vi "Send Finalize View Init.vi"(7 "Priority":T1=enum."Normal" caption="Message Priority (Normal)", 8 "error in (no error)":errorcluster, 10 "View Name":string, 11 "Message Enqueuer in":refnum<class "Message Enqueuer.lvclass">) -> (0 "error out":errorcluster, 3 "Message Enqueuer out":refnum<class "Message Enqueuer.lvclass">)   [LabVIEW 2023, in "Event Actors.lvlib" / "Finalize View Init Msg.lvclass"]
doc: "Sends the <b>Event Actors.lvlib:Finalize View Init Msg.lvclass</b> message.\n\nThis message will call <b>Finalize View Init.vi</b> on the <b>Event Actors.lvlib:Controller Actor.lvclass</b> actor.\n\n<b>Finalize View Init.vi Description</b>\nOverride this method to finalize Views' initialization by generating Controller events to the View specified in the \"View Name\" input terminal. To this end you can call the method \"Generate Event to View\". A typical use case is that of generating Controller events to update the Views upon init about the current state of the Controller."
uses:
  Finalize View Init Msg.lvclass
  Finalize View Init Msg.lvclass/Finalize View Init Msg.ctl
  <vilib>/ActorFramework/Message Enqueuer/Message Enqueuer.lvclass
  C:/Program Files/National Instruments/LabVIEW 2023/vi.lib/ActorFramework/Message/Message.lvclass
  C:/Projects/Shared Libraries/Event Actors/Controller Actor Messages/Finalize View Init Msg/Finalize View Init Msg.lvclass
  <vilib>/ActorFramework/Message Enqueuer/Message Priority.ctl
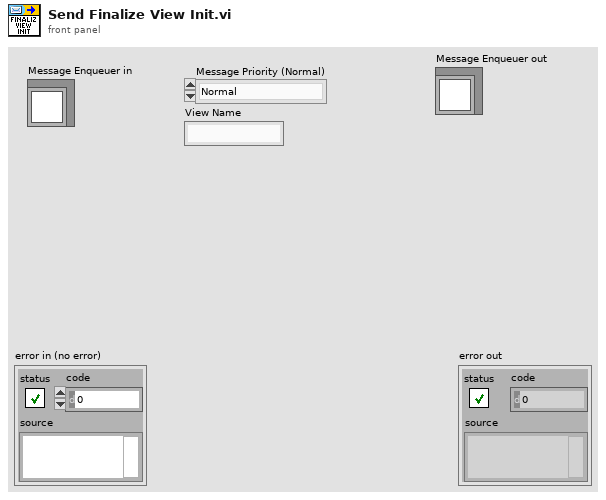
[diagram p1: front panel]
types:
  T1 = typedef "Actor Framework.lvlib/Message Enqueuer.lvclass/Message Priority.ctl" = enum16{"Low", "Normal", "High"}
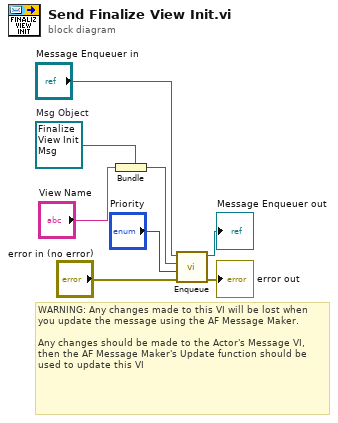
[diagram p0: block diagram]
diagram:
  w7 = refnum<class "Finalize View Init Msg.lvclass"> refnum  # Msg Object
  # "WARNING: Any changes made to this VI will be lost when you update the message using the AF Message Maker.\n\nAny changes should be made to the Actor's Message VI, then the AF Message Maker's Update function should be used to update this VI"
  n1 = Bundle(cluster=w7, "View Name") -> (w2:refnum<class "Finalize View Init Msg.lvclass">)
  n2 = call <vilib>:"Enqueue.vi"("error in (no error)"="error in (no error)", "Message Priority (Normal)"="Priority", "Message"=w2, "Message Enqueuer in"="Message Enqueuer in") -> ("error out"=→"error out":errorcluster, "Message Enqueuer out"=→"Message Enqueuer out":refnum<class "Message Enqueuer.lvclass">)  [unwired: 6 in]
